vi "Set.vi"(8 "error in (no error)":errorcluster, 10 "Variant":variant, 11 "Variant DVR in":refnum<data-value>) -> (0 "error out":errorcluster, 1 "Success?":bool, 3 "Variant DVR out":refnum<data-value>)   [LabVIEW 2019, in "Variant Attributes.lvlib"]
doc: "Sets the variant inside the inside the variant attribute DVR to the input."
uses:
  Variant Attributes.lvlib
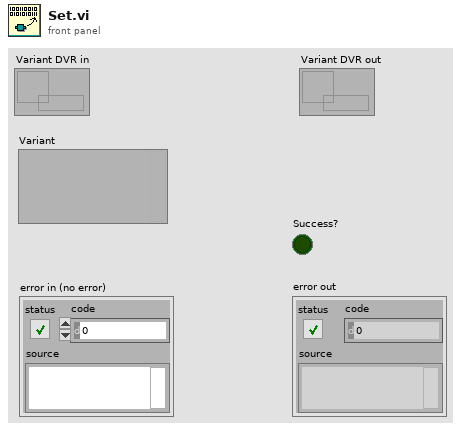
[diagram p1: front panel]
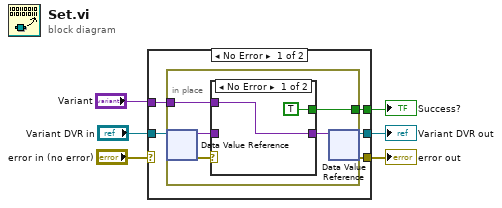
[diagram p0: block diagram]
diagram:
  n1 = case shown="No Error" "error in (no error)" {
    selector: "error in (no error)" -> [_ w20]
    tunnel: "Variant DVR in" -> [w11 w21]
    tunnel: [w10 w21] -> w2
    tunnel: "Variant" -> [w9 _]
    tunnel: [w8 w20] -> w3
    tunnel: [w7 _] -> w1
    frame No Error {
      n2 = in-place {
        in-place-border: w9 -> [w14]
        in-place-border: [w12] -> w7
        n3 = in-place-dvr #1(w11) -> (w16:variant, w15:errorcluster)
        n4 = case shown="No Error" w15 {
          tunnel: w16 -> [_ w19]
          tunnel: w14 -> [w18 _]
          tunnel: [w18 w19] -> w13
          tunnel: [TRUE _] -> w12
          frame No Error {
          }
          frame Error {
          }
        }
        n5 = in-place-dvr #1(w13) -> (w10:refnum<data-value>, w8:errorcluster)
      }
    }
    frame Error {
    }
  }
  "error out" <- w3
  "Variant DVR out" <- w2
  "Success?" <- w1
